vi "Write to Text File and Read from Text File.vi"() -> ()   [LabVIEW 2014]
doc: "This example shows how the Write to Text File and Read from Text File functions operate using different options."
panel:
  out "resulting string":string
  out "remaining string":string
  out "appended path":path
  in  "Path":path
  out "folder names":string[](array[string])
  out "filenames":string[](array[string])
  in  "file path (use dialog)":path
  out "error out":errorcluster
  out "Read Text":string="\n"
  in  "Write Text":string="Line 1 of Text File.\nLine 2 of Text File.\nLine 3 of Text File."
  in  "Operation":u16(ring) items=["Input File as Path", "Input File as Refnum", "Deselecting Convert EOL", "Specifying Read Lines (single line)", "Specifying Read Lines (multiple lines)"]
  # "Overview: Demonstrates the use of the Write to Text File function to write data to a text file, and the Read from Text File function to read data from that text file.\nInstructions:\n1. Specify an Operation to illustrate a particular use case for the Write to Text File and Read from Text File functions.\n2. Run the VI. The 'Write' values below will be written to the file, then read back and displayed in the 'Read' values.\n3. Delete the text file (located at [LabVIEW Data]\\Example Write Read Text File.txt) when you are done."
  # "USB DATA  /media/pi/mwork/Gcode \n\n/srv/chroot/labview"
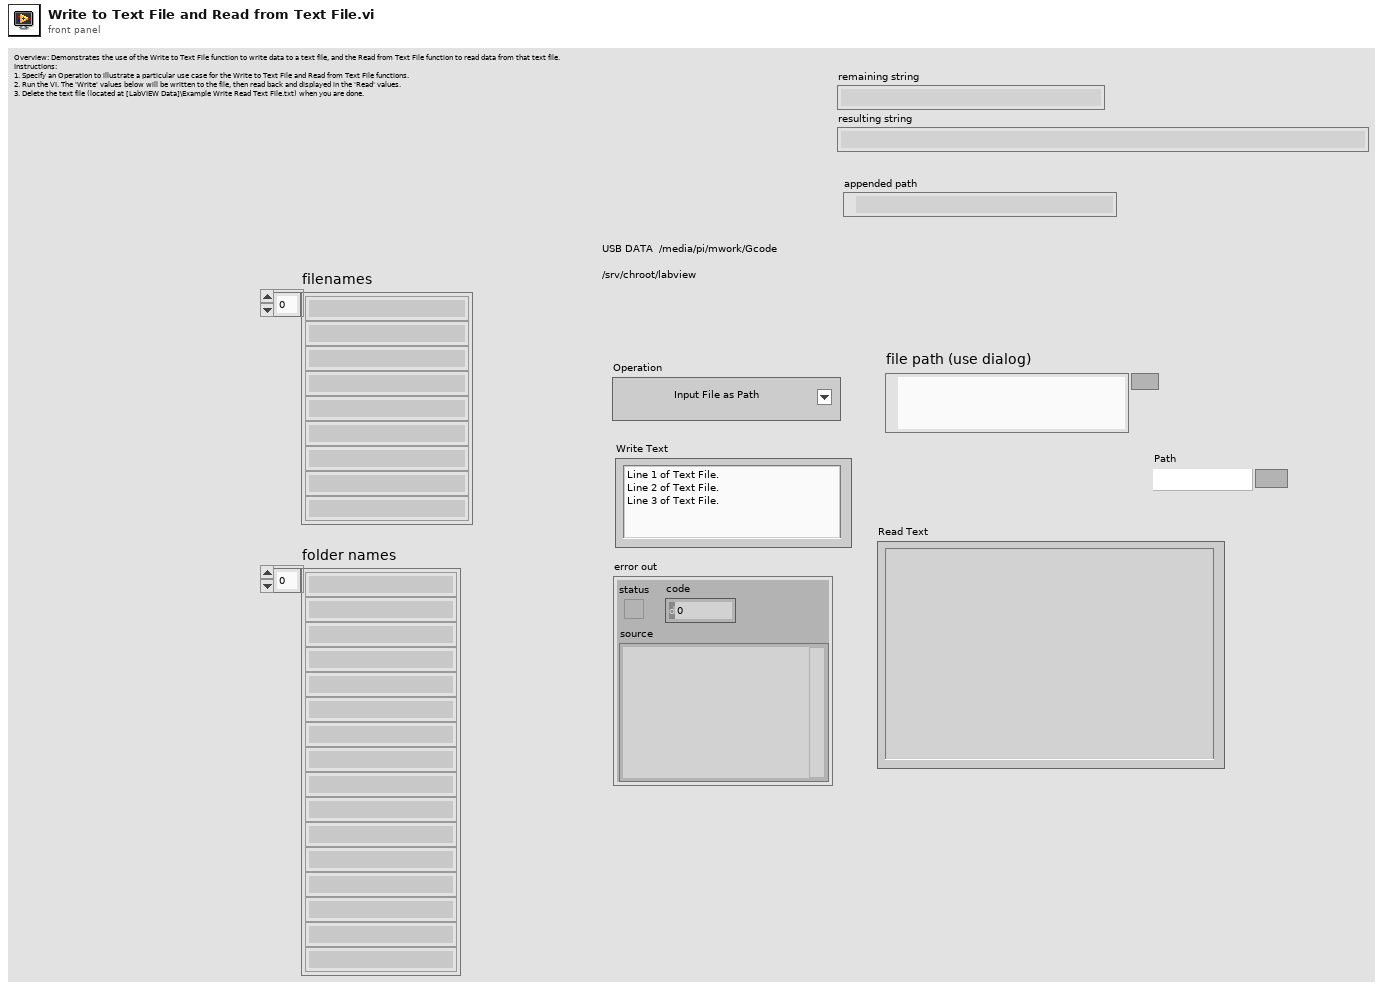
[diagram p1: front panel]
types:
  T1 = enum16{"CheckUSB", "DetachString", "MountUSB", "End"}
  T2 = enum16{"open", "replace", "create", "open or create", "replace or create", "replace or create with confirmation"}
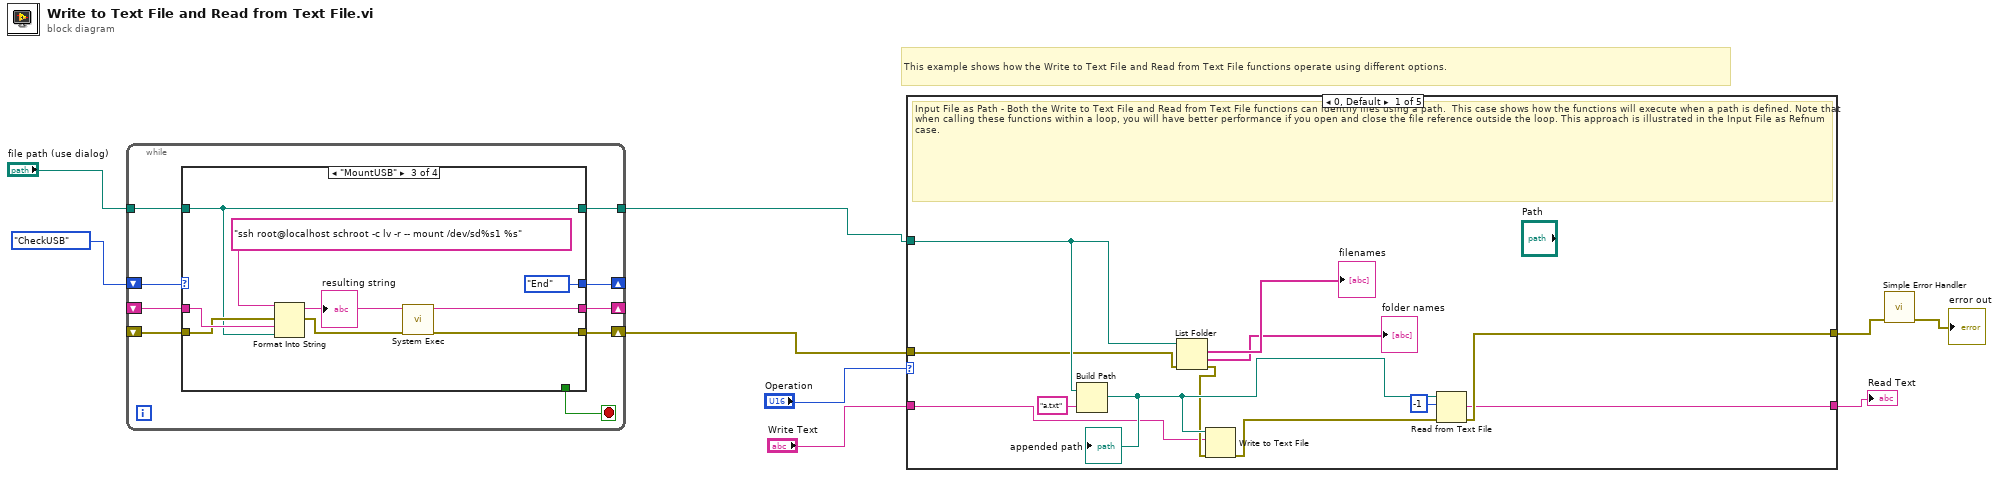
[diagram p0: block diagram]
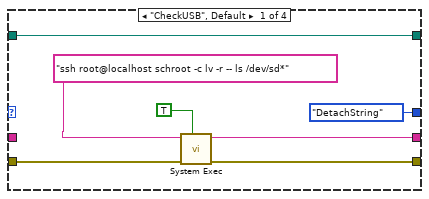
[diagram p2: hidden frame]
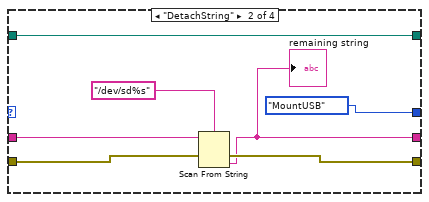
[diagram p3: hidden frame]
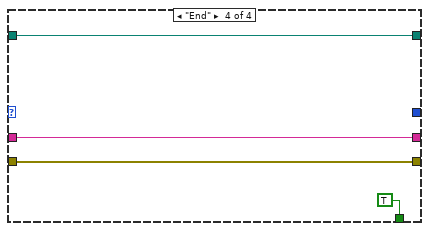
[diagram p4: hidden frame]
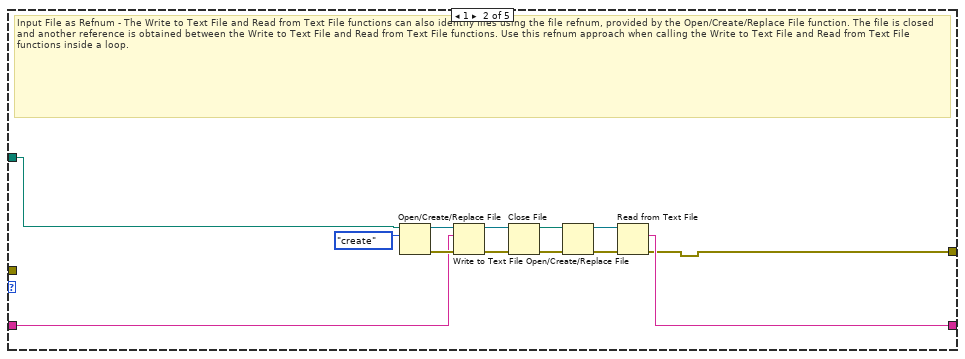
[diagram p5: hidden frame]
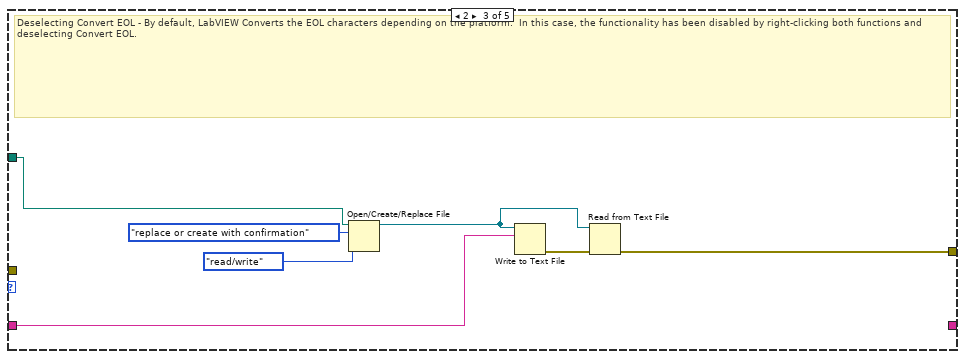
[diagram p6: hidden frame]
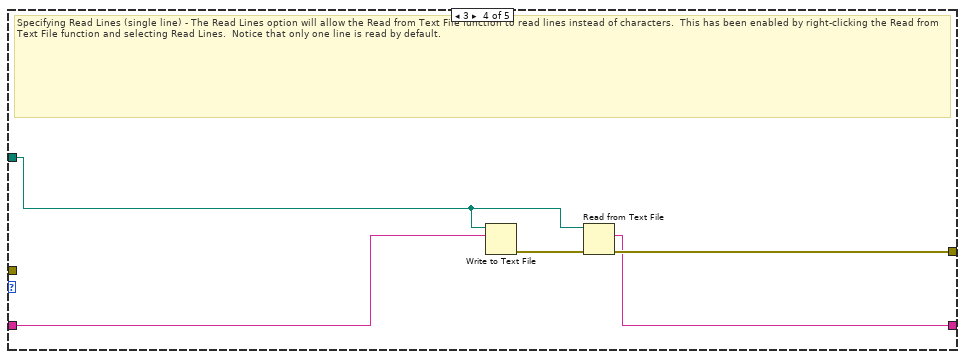
[diagram p7: hidden frame]
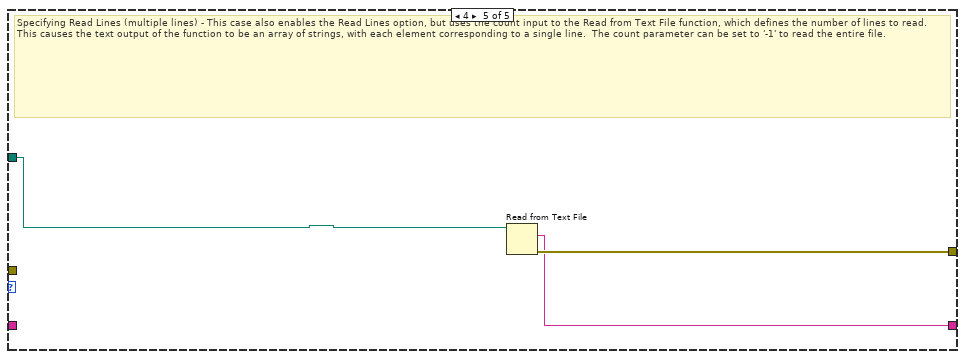
[diagram p8: hidden frame]
diagram:
  # "This example shows how the Write to Text File and Read from Text File functions operate using different options."
  n1 = while {
    shift-right: [w16] -> _
    shift-left: _ -> [w15]
    shift-right: [w13] -> w3
    shift-left: _ -> [w14]
    shift-right: [w12] -> _
    shift-left: T1."CheckUSB" -> [w18]
    tunnel: [w11] -> w2
    tunnel: "file path (use dialog)" -> [w10]
    stop <- w17 stop-if-true
    n2 = case shown="\"MountUSB\"" w18 {
      tunnel: [_ _ _ TRUE] -> w17
      tunnel: [w25 w27 w34 w43] -> w16
      tunnel: w15 -> [_ w32 w40 w43]
      tunnel: w14 -> [w23 w31 w39 w44]
      tunnel: [w22 w30 w35 w44] -> w13
      tunnel: [T1."DetachString" T1."MountUSB" T1."End" _] -> w12
      tunnel: [w19 w26 w33 w42] -> w11
      tunnel: w10 -> [w19 w26 w33 w42]
      frame "CheckUSB", Default {
        n3 = call <vilib>:"System Exec.vi"("wait until completion? (T)"=TRUE, "error in (no error)"=w23, "command line"="ssh root@localhost schroot -c lv -r -- ls /dev/sd*") -> ("error out"=w22:errorcluster, "standard output"=w25:string)  [unwired: 5 in, 2 out]
      }
      frame "DetachString" {
        n4 = Scan From String(format string="/dev/sd%s", input string=w32, error in=w31) -> (error out=w30:errorcluster, output 1=w27:string)  [unwired: 2 in, 2 out]
        "remaining string" <- w27
      }
      frame "MountUSB" {
        n5 = Format Into String(format string="ssh root@localhost schroot -c lv -r -- mount /dev/sd%s1 %s", error in=w39, w40, w33) -> (resulting string=w37:string, error out=w36:errorcluster)  [unwired: 1 in]
        "resulting string" <- w37
        n6 = call <vilib>:"System Exec.vi"("error in (no error)"=w36, "command line"=w37) -> ("error out"=w35:errorcluster, "standard output"=w34:string)  [unwired: 6 in, 2 out]
      }
      frame "End" {
      }
    }
  }
  n7 = case shown="0, Default" "Operation" {
    tunnel: [w55 w59 w76 w81 w85] -> w7
    tunnel: "Write Text" -> [w46 w61 w75 w80 _]
    tunnel: [w51 w60 _ w79 w83] -> w5
    tunnel: w2 -> [w54 w58 w71 w78 w84]
    tunnel: w3 -> [w52 _ _ _ _]
    frame 0, Default {
      # "Input File as Path - Both the Write to Text File and Read from Text File functions can identify files using a path.  This case shows how the functions will execute when a path is defined. Note that when calling these functions within a loop, you will have better performance if you open and close the file reference outside the loop. This approach is illustrated in the Input File as Refnum case."
      n8 = Build Path(base path=w54, name or relative path="a.txt") -> (appended path=w49:path)
      "appended path" <- w49
      n9 = List Folder(path=w54, error in=w52) -> (filenames=→"filenames":string[], folder names=→"folder names":string[], error out=w48:errorcluster)  [unwired: 2 in, 1 out]
      n10 = Write to Text File(file (use dialog)=w49, text=w46, error in=w48) -> (error out=w47:errorcluster)  [unwired: 1 in, 2 out]
      n11 = Read from Text File(file (use dialog)=w49, count=-1, error in=w47) -> (text=w51:string, error out=w55:errorcluster)  [unwired: 1 in, 2 out]
    }
    frame 1 {
      # "Input File as Refnum - The Write to Text File and Read from Text File functions can also identify files using the file refnum, provided by the Open/Create/Replace File function. The file is closed and another reference is obtained between the Write to Text File and Read from Text File functions. Use this refnum approach when calling the Write to Text File and Read from Text File functions inside a loop."
      n12 = Open/Create/Replace File(file path (use dialog)=w58, operation (0:open)=T2."create") -> (refnum out=w68:refnum<file>, error out=w70:errorcluster)  [unwired: 4 in, 1 out]
      n13 = Write to Text File(file (use dialog)=w68, text=w61, error in=w70) -> (refnum out=w67:refnum<file>, error out=w63:errorcluster)  [unwired: 1 in, 1 out]
      n14 = Close File(refnum=w67, error in=w63) -> (path=w66:path, error out=w65:errorcluster)
      n15 = Open/Create/Replace File(file path (use dialog)=w66, error in=w65) -> (refnum out=w64:refnum<file>, error out=w62:errorcluster)  [unwired: 4 in, 1 out]
      n16 = Read from Text File(file (use dialog)=w64, error in=w62) -> (text=w60:string, error out=w59:errorcluster)  [unwired: 2 in, 2 out]
    }
    frame 2 {
      # "Deselecting Convert EOL - By default, LabVIEW Converts the EOL characters depending on the platform.  In this case, the functionality has been disabled by right-clicking both functions and deselecting Convert EOL."
      n17 = Open/Create/Replace File(file path (use dialog)=w71, operation (0:open)=T2."replace or create with confirmation", access (0:read/write)=enum16{"read/write", "read-only", "write-only"}."read/write") -> (refnum out=w74:refnum<file>)  [unwired: 3 in, 2 out]
      n18 = Write to Text File(file (use dialog)=w74, text=w75) -> (error out=w77:errorcluster)  [unwired: 2 in, 2 out]
      n19 = Read from Text File(file (use dialog)=w74, error in=w77) -> (error out=w76:errorcluster)  [unwired: 2 in, 3 out]
    }
    frame 3 {
      # "Specifying Read Lines (single line) - The Read Lines option will allow the Read from Text File function to read lines instead of characters.  This has been enabled by right-clicking the Read from Text File function and selecting Read Lines.  Notice that only one line is read by default."
      n20 = Write to Text File(file (use dialog)=w78, text=w80) -> (error out=w82:errorcluster)  [unwired: 2 in, 2 out]
      n21 = Read from Text File(file (use dialog)=w78, error in=w82) -> (text=w79:string, error out=w81:errorcluster)  [unwired: 2 in, 2 out]
    }
    frame 4 {
      # "Specifying Read Lines (multiple lines) - This case also enables the Read Lines option, but uses the count input to the Read from Text File function, which defines the number of lines to read. This causes the text output of the function to be an array of strings, with each element corresponding to a single line.  The count parameter can be set to '-1' to read the entire file."
      n22 = Read from Text File(file (use dialog)=w84) -> (text=w83:string, error out=w85:errorcluster)  [unwired: 3 in, 2 out]
    }
  }
  "Read Text" <- w5
  n23 = call <vilib>:"Simple Error Handler.vi"("error in (no error)"=w7) -> ("error out"=→"error out":errorcluster)  [unwired: 4 in, 4 out]
